vi "SMU Switch Handshaking - Advanced - DMM.vi"(4 "Source:Advanced:Source Delay":dbl=4e-05 format="%#_6p", 5 "Source:Transient Response":i32(ring)=1039 items=["Slow"=1041, "Normal"=1038, "Fast"=1039, "Custom"=1042], 7 "Measurement:Sense":i32(ring)=1008 items=["Local"=1008, "Remote"=1009], 8 "channels":string="0", 9 "Current":dbl=0.4 format="%#_6p", 10 "Voltage":dbl=0.6 format="%#_6p", 11 "resource name":refnum<k15>="SMU" caption="SMU resource name") -> ()   [LabVIEW 2019]
uses:
  <instrlib>/niSwitch/niSwitch.llb/niSwitch Topologies.ctl
  <instrlib>/niSwitch/niSwitch.llb/niSwitch Trigger Input.ctl
  <instrlib>/niSwitch/niSwitch.llb/niSwitch Scan Advanced Output.ctl
  <instrlib>/niDMM/nidmm.llb/niDMM Function.ctl
  <instrlib>/niDMM/nidmm.llb/niDMM Trigger.ctl
  <instrlib>/niDMM/nidmm.llb/niDMM Slope.ctl
  <instrlib>/niDCPower/nidcpower.llb/niDCPower Export Signal - Signal.ctl
  <instrlib>/niDMM/nidmm.llb/niDMM Sample Trigger.ctl
  <instrlib>/niDMM/nidmm.llb/niDMM Control Actions.ctl
  <instrlib>/niDCPower/nidcpower.llb/niDCPower Wait For Event - Event.ctl
  <instrlib>/niDCPower/nidcpower.llb/niDCPower Configure Digital Edge Start Trigger.vi
  <instrlib>/niDCPower/nidcpower.llb/niDCPower Configure Digital Edge Sequence Advance Trigger.vi
  <instrlib>/niDMM/nidmm.llb/niDMM Configure Measurement Absolute.vi
  <vilib>/ptbypt/NI_PtbyPt.lvlib
panel:
  out "R ch5":dbl=2.5910331699131763e-06 format="%#_8p"
  out "Waveform Chart ch5":dbl(graph)=2.5910331699131763e-06
  out "standard deviation ch5":dbl=1.2903874661428992e-07 format="%.6p"
  out "R ch2":dbl=7.972830555761924e-07 format="%#_8p"
  out "Waveform Chart ch2":dbl(graph)=7.972830555761924e-07
  out "standard deviation ch2":dbl=2.4873144111684715e-07 format="%.6p"
  out "R ch4":dbl=4.337850347432063e-06 format="%#_8p"
  out "Waveform Chart ch4":dbl(graph)=4.337850347432063e-06
  out "standard deviation ch4":dbl=1.3349477799504632e-07 format="%.6p"
  out "R ch1":dbl=1.766350792285936e-06 format="%#_8p"
  out "Waveform Chart ch1":dbl(graph)=1.766350792285936e-06
  out "standard deviation ch1":dbl=1.0073898391211356e-07 format="%.6p"
  out "R ch3":dbl=nan format="%#_8p"
  out "Waveform Chart ch3":dbl(graph)=nan
  out "standard deviation ch3":dbl=nan format="%.6p"
  out "standard deviation ch0":dbl=9.036112711225856e-08 format="%.6p"
  out "Waveform Chart ch0":dbl(graph)=2.086031872229756e-06
  out "R ch0":dbl=2.086031872229756e-06 format="%#_8p"
  out "voltage measurements":dbl[](array[numeric])=[1.0598444973016901e-05, 1.0214343256868734e-05, 1.0841159071034221e-05]
  in  "Configuration:Advanced:Number Of Averages":i32=1
  in  "Configuration:Advanced:Aperture Time":dbl=0.05
  in  "Configuration:Advanced:Aperture Time Units":i32(ring) items=["Seconds", "Power Line Cycles"]
  in  "Device Name":refnum<k15>="4082"
  in  "Slope":T1
  in  "DMM Trigger Source":T2=enum."TTL 2"
  in  "Range":dbl=0.1 format="%.2p"
  in  "Function":T3
  out "Elapsed Time (ms)":u32=9613
  in  "scan advanced output (External)":T4=enum."TTL1" caption="Scan Advanced Destination"
  in  "Trigger Source":T5=enum."TTL0"
  in  "topology name":T6="2530/1-Wire 4x32 Matrix" caption="Topology Name"
  in  "scan list":string="r0->c0&r1->c1&r2->c2&r3->c3;\nr0->c4&r1->c5&r2->c6&r3->c7;\nr0->c8&r1->c9&r2->c10&r3->c11;\nr0->c12&r1->c13&r2->c14&r3->c15;\nr0->c16&r1->c17&r2->c18&r3->c19;\nr0->c20&r1->c21&r2->c22&r3->c23;\n\n" caption="Scan List"
  in  "resource name 2":refnum<k15>="PXI1Slot5" caption="Switch Resource Name"
  in  "Measurement:Aperture Time":dbl=0.08333333 format="%#_6p"
  out "error out":errorcluster={"status"=FALSE, "code"=1073356801, "source"="niDMM Fetch Multi Point.vi<ERR>Over range.\n\n "}
  out "current measurements":dbl[](array[numeric])=[0.24066338808611681, -0.24109991223961136, -3.355526367182504e-08]
  in  "Measurement:Advanced:DC Noise Rejection":i32(ring)=1044 items=["Normal"=1044, "Second-Order"=1043]
  in  "Source:Advanced:Sequence Loop Count":i32=39
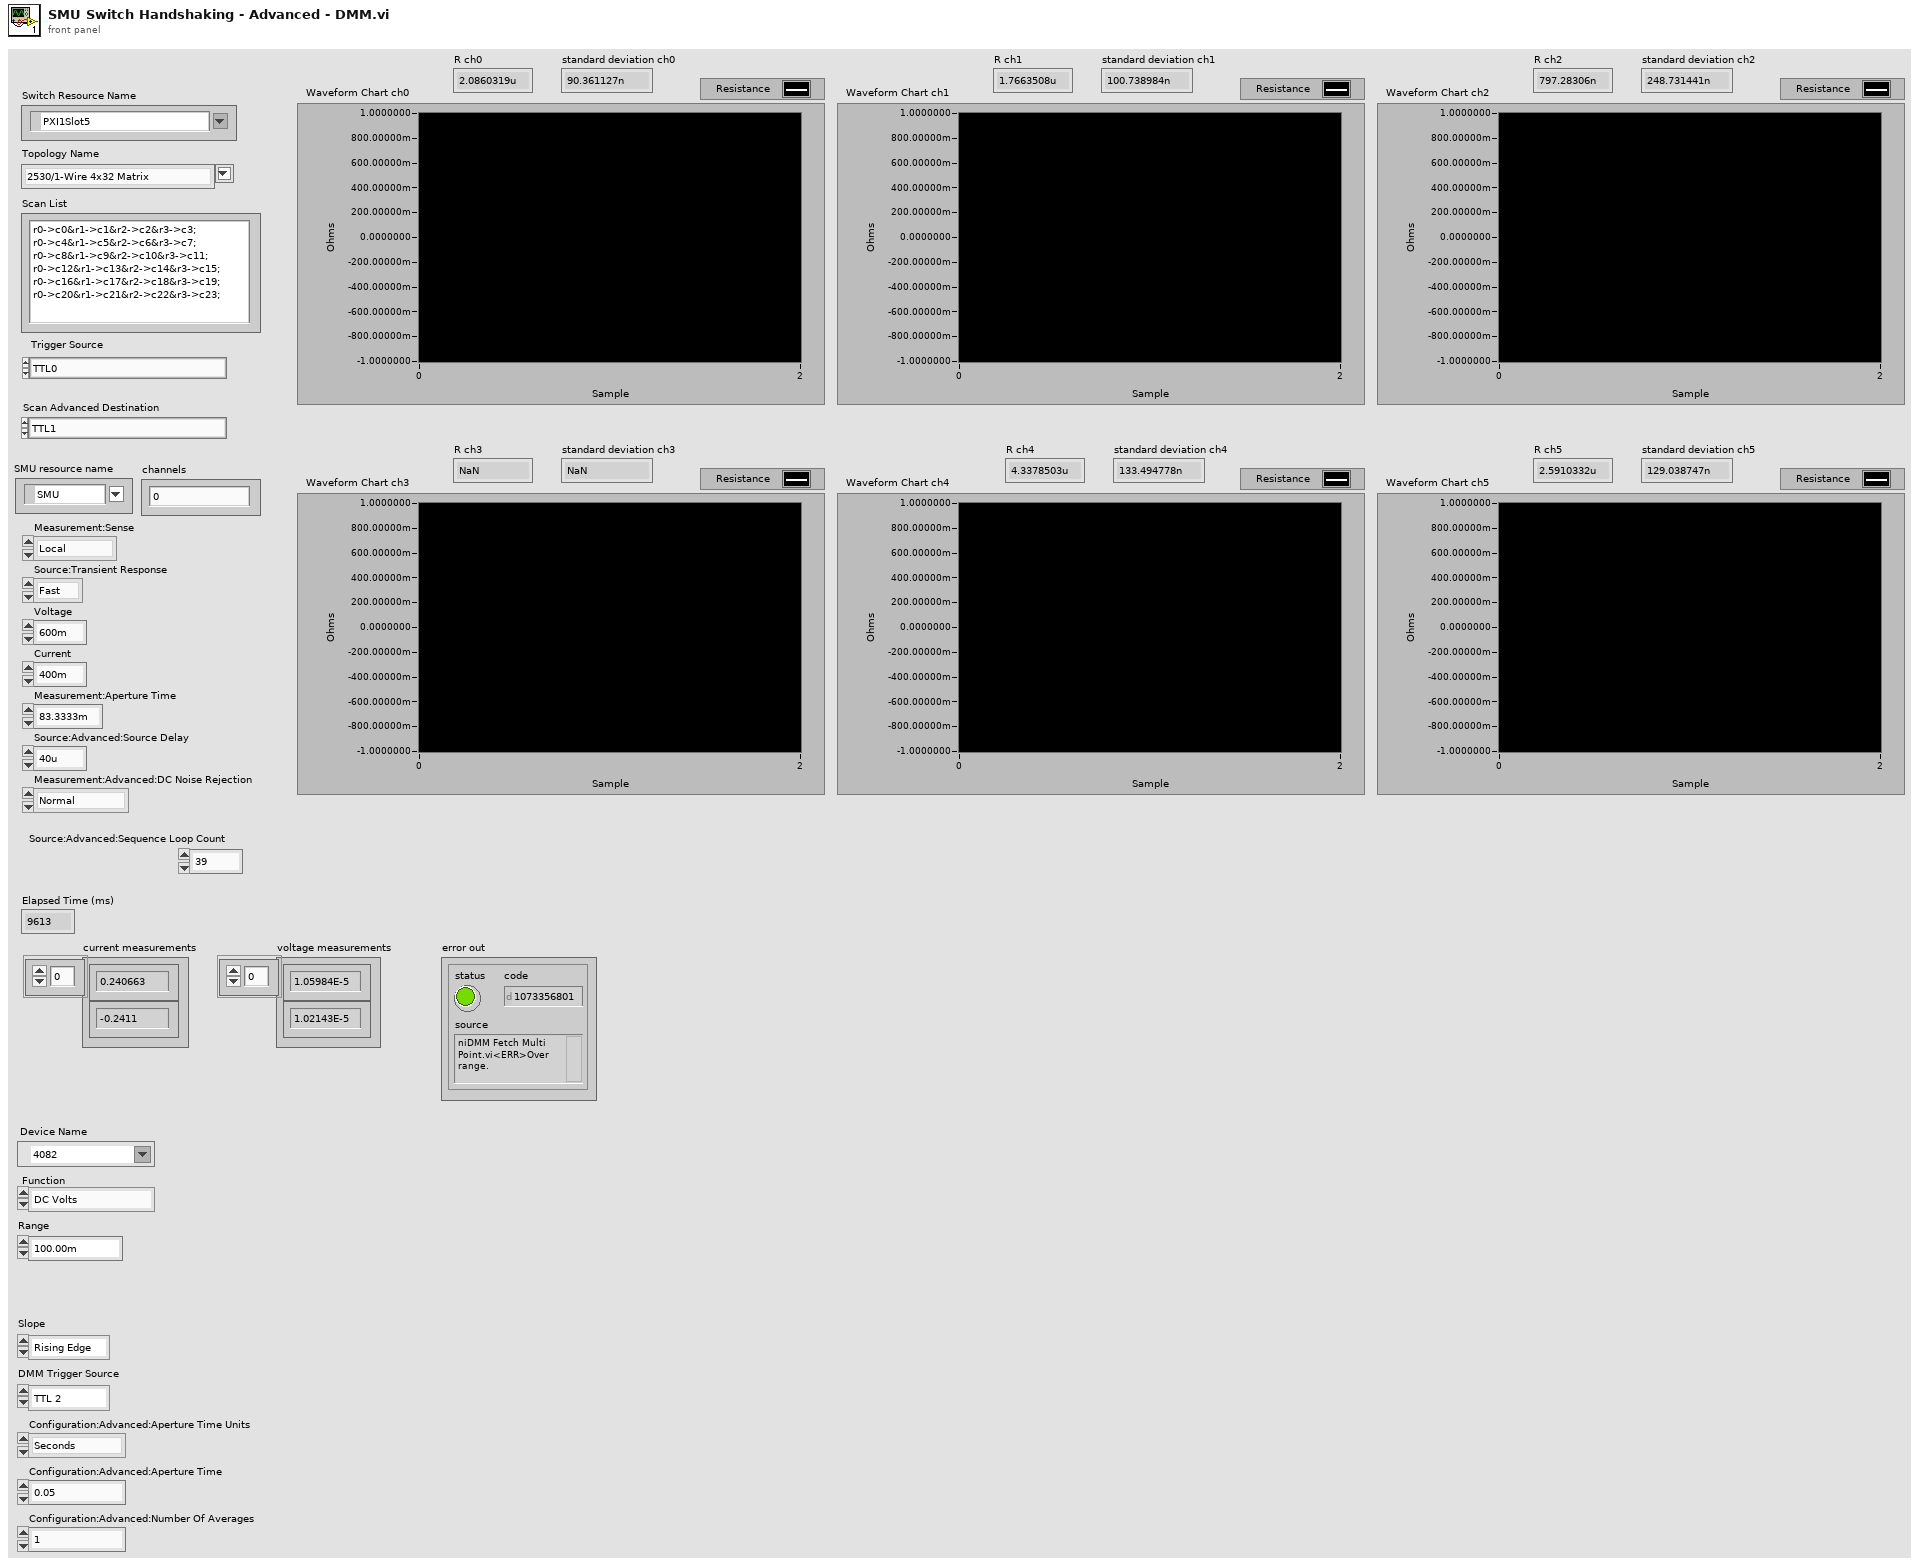
[diagram p1: front panel]
types:
  T1 = typedef "niDMM Slope.ctl" = enum16{"Rising Edge", "Falling Edge"}
  T2 = typedef "niDMM Trigger.ctl" = enum16{"Immediate", "External", "TTL 0", "TTL 1", "TTL 2", "TTL 3", "TTL 4", "TTL 5", "TTL 6", "Software", "TTL 7", "PXI Star", "LBR Trig 1", "Aux Trig 1"}
  T3 = typedef "niDMM Function.ctl" = enum16{"DC Volts", "AC Volts", "DC Current", "AC Current", "2-wire Resistance", "4-wire Resistance", "Diode", "Frequency", "Period", "AC Volts DC Coupled", "Capacitance", "Inductance", "Temperature"}
  T4 = typedef "niSwitch Scan Advanced Output.ctl" = enum16{"None", "External", "TTL0", "TTL1", "TTL2", "TTL3", "TTL4", "TTL5", "TTL6", "TTL7", "ECL0", "ECL1", "PXI Star", "Rear Connector", "Front Connector", "Rear Connector Module 1", "Rear Connector Module 2", "Rear Connector Module 3", "Rear Connector Module 4", "Rear Connector Module 5", "Rear Connector Module 6", "Rear Connector Module 7", "Rear Connector Module 8", "Rear Connector Module 9", "Rear Connector Module 10", "Rear Connector Module 11", "Rear Connector Module 12", "Front Connector Module 1", "Front Connector Module 2", "Front Connector Module 3", "Front Connector Module 4", "Front Connector Module 5", "Front Connector Module 6", "Front Connector Module 7", "Front Connector Module 8", "Front Connector Module 9", "Front Connector Module 10", "Front Connector Module 11", "Front Connector Module 12"}
  T5 = typedef "niSwitch Trigger Input.ctl" = enum16{"Immediate", "External", "TTL0", "TTL1", "TTL2", "TTL3", "TTL4", "TTL5", "TTL6", "TTL7", "ECL0", "ECL1", "PXI Star", "Software Trigger Function", "Rear Connector", "Front Connector", "Rear Connector of Module 1", "Rear Connector of Module 2", "Rear Connector of Module 3", "Rear Connector of Module 4", "Rear Connector of Module 5", "Rear Connector of Module 6", "Rear Connector of Module 7", "Rear Connector of Module 8", "Rear Connector of Module 9", "Rear Connector of Module 10", "Rear Connector of Module 11", "Rear Connector of Module 12", "Front Connector of Module 1", "Front Connector of Module 2", "Front Connector of Module 3", "Front Connector of Module 4", "Front Connector of Module 5", "Front Connector of Module 6", "Front Connector of Module 7", "Front Connector of Module 8", "Front Connector of Module 9", "Front Connector of Module 10", "Front Connector of Module 11", "Front Connector of Module 12"}
  T6 = typedef "niSwitch Topologies.ctl" = string
  T7 = typedef "niDCPower Export Signal - Signal.ctl" = i32
  T8 = typedef "niDMM Control Actions.ctl" = i32
  T9 = typedef "niDMM Sample Trigger.ctl" = enum16{"Immediate", "External", "TTL 0", "TTL 1", "TTL 2", "TTL 3", "TTL 4", "TTL 5", "TTL 6", "Interval", "Software", "TTL 7", "PXI Star", "LBR Trig 1", "Aux Trig 1"}
  T10 = typedef "niDCPower Wait For Event - Event.ctl" = i32
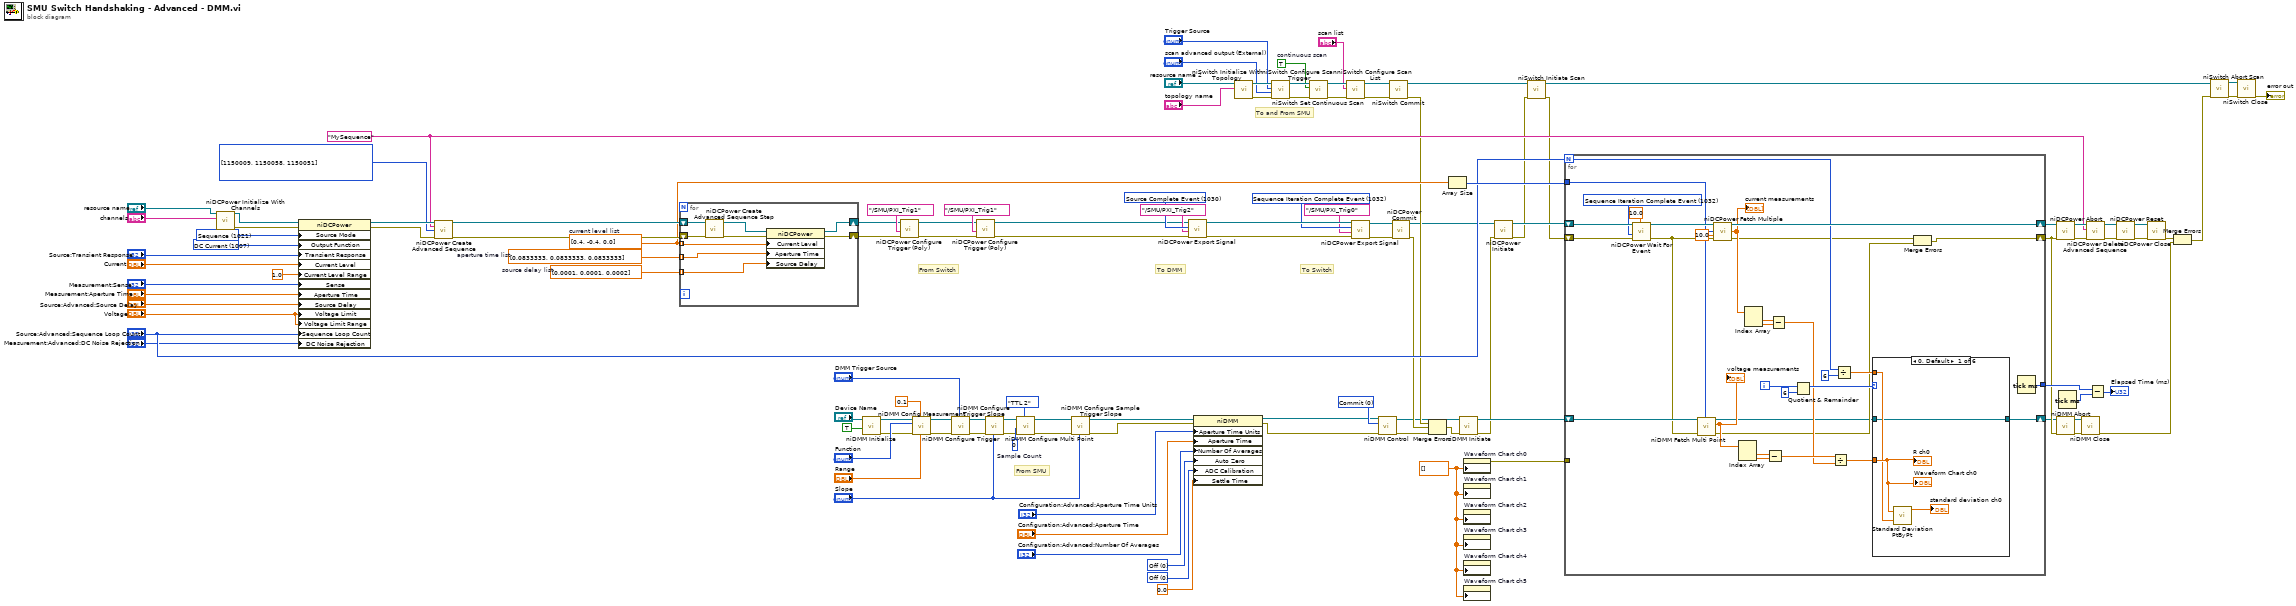
[diagram p0: block diagram]
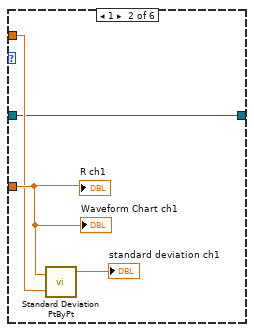
[diagram p2: hidden frame]
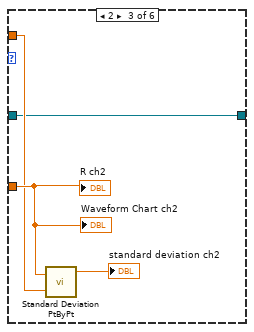
[diagram p3: hidden frame]
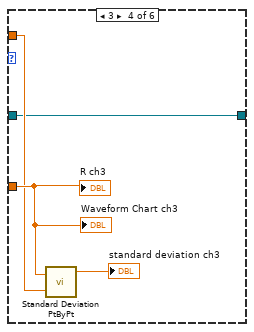
[diagram p4: hidden frame]
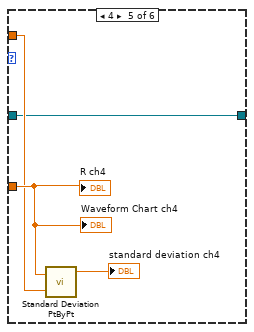
[diagram p5: hidden frame]
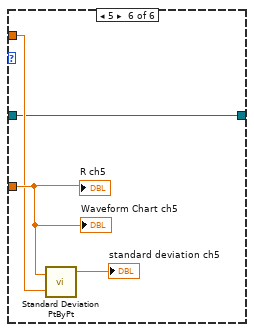
[diagram p6: hidden frame]
diagram:
  w2 = 0 items=["Auto"=-1, "Off"=0, "On"=1] ("Configuration:Measurement Options:ADC Calibration")
  w3 = 0 items=["Auto"=-1, "Off"=0, "On"=1, "Once"=2] ("Configuration:Measurement Options:Auto Zero")
  w7 = T7 1032 items=["Source Complete Event"=1030, "Measure Complete Event"=1031, "Sequence Iteration Complete Event"=1032, "Sequence Engine Done Event"=1033, "Pulse Complete Event"=1051, "Ready For Pulse Trigger Event"=1052, "Start Trigger"=1034, "Source Trigger"=1035, "Measure Trigger"=1036, "Sequence Advance Trigger"=1037, "Pulse Trigger"=1053] ("signal")
  w31 = T8 0 items=["Commit"] ("Control Action")
  w53 = 0  # Sample Count
  w58 = T7 1030 items=["Source Complete Event"=1030, "Measure Complete Event"=1031, "Sequence Iteration Complete Event"=1032, "Sequence Engine Done Event"=1033, "Pulse Complete Event"=1051, "Ready For Pulse Trigger Event"=1052, "Start Trigger"=1034, "Source Trigger"=1035, "Measure Trigger"=1036, "Sequence Advance Trigger"=1037, "Pulse Trigger"=1053] ("signal")
  w61 = dbl[] [0.4, -0.4, 0.0]  # current level list
  w8 = dbl[] [0.0833333, 0.0833333, 0.0833333]  # aperture time list
  w67 = i32[] [1150009, 1150058, 1150051] items=["Source -> Output Function"=1150008, "Source -> Output Enabled"=1250006, "Source -> Output Resistance"=1150061, "Source -> Transient Response"=1150062, "Source -> Custom Transient Response -> Voltage Gain Bandwidth"=1150067, "Source -> Custom Transient Response -> Voltage Compensation Frequency"=1150068, "Source -> Custom Transient Response -> Voltage Pole-Zero Ratio"=1150069, "Source -> Custom Transient Response -> Current Gain Bandwidth"=1150070, "Source -> Custom Transient Response -> Current Compensation Frequency"=1150071, "Source -> Custom Transient Response -> Current Pole-Zero Ratio"=1150072, "Source -> DC Voltage -> Voltage Level"=1250001, "Source -> DC Voltage -> Voltage Level Range"=1150005, "Source -> DC Voltage -> Current Limit"=1250005, "Source -> DC Voltage -> Current Limit High"=1150187, "Source -> DC Voltage -> Current Limit Low"=1150188, "Source -> DC Voltage -> Current Limit Range"=1150004, "Source -> DC Current -> Current Level"=1150009, "Source -> DC Current -> Current Level Range"=1150011, "Source -> DC Current -> Voltage Limit"=1150010, "Source -> DC Current -> Voltage Limit High"=1150185, "Source -> DC Current -> Voltage Limit Low"=1150186, "Source -> DC Current -> Voltage Limit Range"=1150012, "Source -> Pulse Voltage -> Pulse Voltage Level"=1150080, "Source -> Pulse Voltage -> Pulse Bias Voltage Level"=1150082, "Source -> Pulse Voltage -> Pulse Voltage Level Range"=1150084, "Source -> Pulse Voltage -> Pulse Current Limit"=1150081, "Source -> Pulse Voltage -> Pulse Current Limit High"=1150193, "Source -> Pulse Voltage -> Pulse Current Limit Low"=1150194, "Source -> Pulse Voltage -> Pulse Bias Current Limit"=1150083, "Source -> Pulse Voltage -> Pulse Bias Current Limit High"=1150195, "Source -> Pulse Voltage -> Pulse Bias Current Limit Low"=1150196, "Source -> Pulse Voltage -> Pulse Current Limit Range"=1150085, "Source -> Pulse Current -> Pulse Current Level"=1150086, "Source -> Pulse Current -> Pulse Bias Current Level"=1150088, "Source -> Pulse Current -> Pulse Current Level Range"=1150090, "Source -> Pulse Current -> Pulse Voltage Limit"=1150087, "Source -> Pulse Current -> Pulse Voltage Limit High"=1150189, "Source -> Pulse Current -> Pulse Voltage Limit Low"=1150190, "Source -> Pulse Current -> Pulse Bias Voltage Limit"=1150089, "Source -> Pulse Current -> Pulse Bias Voltage Limit High"=1150191, "Source -> Pulse Current -> Pulse Bias Voltage Limit Low"=1150192, "Source -> Pulse Current -> Pulse Voltage Limit Range"=1150091, "Source -> Advanced -> Source Delay"=1150051, "Source -> Advanced -> Pulse Bias Delay"=1150092, "Source -> Advanced -> Pulse On Time"=1150093, "Source -> Advanced -> Pulse Off Time"=1150094, "Source -> Advanced -> OVP Enabled"=1250002, "Source -> Advanced -> OVP Limit"=1250003, "Source -> Advanced -> Compliance Limit Symmetry"=1150184, "Source -> Advanced -> Sequence Step Delta Time"=1150198, "Measurement -> Sense"=1150013, "Measurement -> Aperture Time"=1150058, "Measurement -> Measure Record Length"=1150063, "Measurement -> Advanced -> DC Noise Rejection"=1150066] ("advanced sequence properties")
  w68 = "MySequence" ("sequence name")
  w100 = TRUE  # continuous scan
  w64 = dbl[] [0.0001, 0.0001, 0.0002]  # source delay list
  w11 = dbl[] [] ("History Data")
  w119 = 1007 items=["DC Voltage"=1006, "DC Current"=1007, "Pulse Voltage"=1049, "Pulse Current"=1050] ("Source:Output Function")
  w120 = 1021 items=["Single Point"=1020, "Sequence"=1021] ("Source:Source Mode")
  # "To and From SMU"
  # "From SMU"
  # "To Switch"
  # "To DMM"
  # "From Switch"
  n1 = call <instrlib>:"niDCPower Initialize With Channels.vi"("channels"="channels", "resource name"="resource name") -> ("error out"=w113:errorcluster, "instrument handle out"=w114:refnum<k15>)  [unwired: 8 in]
  n2 = property class="niDCPower"(reference=w114, error in=w113, "Source Mode"=w120, "Output Function"=w119, "Transient Response"="Source:Transient Response", "Current Level"="Current", "Current Level Range"=1.0 ("Source:DC Current:Current Level Range"), "Sense"="Measurement:Sense", "Aperture Time"="Measurement:Aperture Time", "Source Delay"="Source:Advanced:Source Delay", "Voltage Limit"="Voltage", "Voltage Limit Range"="Voltage", "Sequence Loop Count"="Source:Advanced:Sequence Loop Count", "DC Noise Rejection"="Measurement:Advanced:DC Noise Rejection") -> (reference out=w76:refnum<k15>, error out=w75:errorcluster)
  n3 = call <instrlib>:"niDCPower Create Advanced Sequence.vi"("instrument handle"=w76, "sequence name"=w68, "advanced sequence properties"=w67, "error in (no error)"=w75) -> ("instrument handle out"=w66:refnum<k15>, "error out"=w65:errorcluster)  [unwired: 10 in]
  n4 = for {
    shift-right: [w126] -> w62
    shift-left: w65 -> [w129]
    shift-right: [w125] -> w63
    shift-left: w66 -> [w124]
    tunnel: w64 -> [w123] mode=indexing
    tunnel: w61 -> [w121] mode=indexing
    tunnel: w8 -> [w122] mode=indexing
    n5 = call <instrlib>:"niDCPower Create Advanced Sequence Step.vi"("error in (no error)"=w129, "instrument handle"=w124) -> ("error out"=w127:errorcluster, "instrument handle out"=w128:refnum<k15>)  [unwired: 8 in]
    n6 = property class="niDCPower"(reference=w128, error in=w127, "Current Level"=w121, "Aperture Time"=w122, "Source Delay"=w123) -> (reference out=w125:refnum<k15>, error out=w126:errorcluster)
  }
  n7 = call <instrlib>:"niDMM Initialize.vi"("Reset"=TRUE, "Instrument Descriptor"="Device Name") -> ("error out"=w39:errorcluster, "instrument handle out"=w38:refnum<k15>)  [unwired: 8 in]
  n8 = call-poly <instrlib>:"niDCPower Configure Trigger (Poly).vi"("error in (no error)"=w62, "input terminal"=tag "/SMU/PXI_Trig1", "instrument handle"=w63) -> ("error out"=w81:errorcluster, "instrument handle out"=w82:refnum<k15>)  [unwired: 7 in]
  n9 = call-poly <instrlib>:"niDMM Config Measurement.vi"("Range"="Range", "Resolution"=0.1, "error in (no error)"=w39, "Function"="Function", "instrument handle"=w38) -> ("error out"=w45:errorcluster, "instrument handle out"=w44:refnum<k15>)  [unwired: 5 in]
  n10 = call <instrlib>:"niDMM Configure Trigger.vi"("Trigger Source"="DMM Trigger Source", "error in (no error)"=w45, "instrument handle"=w44) -> ("error out"=w47:errorcluster, "instrument handle out"=w46:refnum<k15>)  [unwired: 7 in]
  n11 = call-poly <instrlib>:"niDCPower Configure Trigger (Poly).vi"("error in (no error)"=w81, "input terminal"=tag "/SMU/PXI_Trig1", "instrument handle"=w82) -> ("error out"=w9:errorcluster, "instrument handle out"=w10:refnum<k15>)  [unwired: 7 in]
  n12 = call <instrlib>:"niDMM Configure Trigger Slope.vi"("Slope"="Slope", "error in (no error)"=w47, "instrument handle"=w46) -> ("error out"=w49:errorcluster, "instrument handle out"=w48:refnum<k15>)  [unwired: 7 in]
  n13 = call <instrlib>:"niDMM Configure Multi Point.vi"("Sample Trigger"=niDMM_Sample_Trigger."TTL 2", "error in (no error)"=w49, "Sample Count"=w53, "instrument handle"=w48) -> ("error out"=w51:errorcluster, "instrument handle out"=w50:refnum<k15>)  [unwired: 6 in]
  n14 = call <instrlib>:"niDMM Configure Sample Trigger Slope.vi"("Slope"="Slope", "error in (no error)"=w51, "instrument handle"=w50) -> ("error out"=w22:errorcluster, "instrument handle out"=w23:refnum<k15>)  [unwired: 7 in]
  n15 = call <instrlib>:"niDCPower Export Signal.vi"("error in (no error)"=w9, "output terminal"=tag "/SMU/PXI_Trig2", "signal"=w58, "instrument handle"=w10) -> ("error out"=w59:errorcluster, "instrument handle out"=w60:refnum<k15>)  [unwired: 6 in]
  n16 = property class="niDMM"(reference=w23, error in=w22, "Aperture Time Units"="Configuration:Advanced:Aperture Time Units", "Aperture Time"="Configuration:Advanced:Aperture Time", "Number Of Averages"="Configuration:Advanced:Number Of Averages", "Auto Zero"=w3, "ADC Calibration"=w2, "Settle Time"=0.0 ("Configuration:Advanced:Settle Time")) -> (reference out=w13:refnum<k15>, error out=w12:errorcluster)
  n17 = call <instrlib>:"niSwitch Initialize With Topology.vi"("topology name"="topology name", "resource name"="resource name 2") -> ("error out"=w97:errorcluster, "instrument handle out"=w98:refnum<k15>)  [unwired: 3 in, 5 out]
  n18 = call <instrlib>:"niSwitch Configure Scan Trigger.vi"("error in (no error)"=w97, "scan advanced output (External)"="scan advanced output (External)", "trigger input (External)"="Trigger Source", "instrument handle"=w98) -> ("error out"=w101:errorcluster, "instrument handle out"=w103:refnum<k15>)  [unwired: 1 in, 5 out]
  n19 = call <instrlib>:"niSwitch Set Continuous Scan.vi"("error in (no error)"=w101, "continuous scan (False)"=w100, "instrument handle"=w103) -> ("error out"=w95:errorcluster, "instrument handle out"=w96:refnum<k15>)  [unwired: 7 out]
  n20 = call <instrlib>:"niSwitch Configure Scan List.vi"("error in (no error)"=w95, "scan list"="scan list", "instrument handle"=w96) -> ("error out"=w92:errorcluster, "instrument handle out"=w91:refnum<k15>)  [unwired: 1 in, 6 out]
  n21 = call <instrlib>:"niDCPower Export Signal.vi"("error in (no error)"=w59, "output terminal"=tag "/SMU/PXI_Trig0", "signal"=w7, "instrument handle"=w60) -> ("error out"=w34:errorcluster, "instrument handle out"=w35:refnum<k15>)  [unwired: 6 in]
  n22 = call <instrlib>:"niDMM Control.vi"("error in (no error)"=w12, "Control Action"=w31, "instrument handle"=w13) -> ("error out"=w30:errorcluster, "instrument handle out"=w24:refnum<k15>)  [unwired: 7 in]
  n23 = call <instrlib>:"niSwitch Commit.vi"("error in (no error)"=w92, "instrument handle"=w91) -> ("error out"=w33:errorcluster, "instrument handle out"=w90:refnum<k15>)  [unwired: 8 out]
  n24 = call <instrlib>:"niDCPower Commit.vi"("error in (no error)"=w34, "instrument handle"=w35) -> ("error out"=w32:errorcluster, "instrument handle out"=w27:refnum<k15>)  [unwired: 8 in]
  n25 = Merge Errors(w33, w32, w30) -> (w29:errorcluster)
  n26 = Array Size(array=w61) -> (size(s)=w115:i32)
  n27 = call <instrlib>:"niDMM Initiate.vi"("error in (no error)"=w29, "instrument handle"=w24) -> ("error out"=w28:errorcluster, "instrument handle out"=w36:refnum<k15>)  [unwired: 8 in]
  n28 = property on="Waveform Chart ch0" class="WFChart (strict)"("History Data"=w11) -> (error out=w5:errorcluster)  [unwired: 2 in, 1 out]
  n29 = property on="Waveform Chart ch1" class="WFChart (strict)"("History Data"=w11) -> ()  [unwired: 2 in, 2 out]
  n30 = property on="Waveform Chart ch2" class="WFChart (strict)"("History Data"=w11) -> ()  [unwired: 2 in, 2 out]
  n31 = property on="Waveform Chart ch3" class="WFChart (strict)"("History Data"=w11) -> ()  [unwired: 2 in, 2 out]
  n32 = property on="Waveform Chart ch4" class="WFChart (strict)"("History Data"=w11) -> ()  [unwired: 2 in, 2 out]
  n33 = property on="Waveform Chart ch5" class="WFChart (strict)"("History Data"=w11) -> ()  [unwired: 2 in, 2 out]
  n34 = call <instrlib>:"niDCPower Initiate.vi"("error in (no error)"=w28, "instrument handle"=w27) -> ("error out"=w26:errorcluster, "instrument handle out"=w104:refnum<k15>)  [unwired: 8 in]
  n35 = call <instrlib>:"niSwitch Initiate Scan.vi"("error in (no error)"=w26, "instrument handle"=w90) -> ("error out"=w25:errorcluster, "instrument handle out"=w93:refnum<k15>)  [unwired: 8 out]
  n36 = for {
    N: "Source:Advanced:Sequence Loop Count" -> [w149]
    tunnel: w115 -> [w143]
    shift-right: [w134] -> w18
    shift-left: w25 -> [w145]
    shift-right: [w156] -> w108
    shift-left: w104 -> [w160]
    tunnel: w5 -> [_]
    tunnel: [w153] -> w80
    shift-right: [w132] -> w14
    shift-left: w36 -> [w144]
    i -> [w152]
    w159 = T10 1032 items=["Source Complete Event"=1030, "Measure Complete Event"=1031, "Sequence Iteration Complete Event"=1032, "Sequence Engine Done Event"=1033, "Pulse Complete Event"=1051, "Ready For Pulse Trigger Event"=1052] ("event")
    n37 = call <instrlib>:"niDCPower Wait For Event.vi"("timeout (sec)"=10.0, "error in (no error)"=w145, "event"=w159, "instrument handle"=w160) -> ("error out"=w131:errorcluster, "instrument handle out"=w157:refnum<k15>)  [unwired: 6 in]
    n38 = call <instrlib>:"niDMM Fetch Multi Point.vi"("Number to Fetch"=w143, "error in (no error)"=w131, "instrument handle"=w144) -> ("error out"=w135:errorcluster, "Measurements"=w137:dbl[], "instrument handle out"=w133:refnum<k15>)  [unwired: 5 in, 1 out]
    "voltage measurements" <- w137
    n39 = call <instrlib>:"niDCPower Fetch Multiple.vi"("instrument handle"=w157, "count (1)"=w143, "timeout (sec)"=10.0, "error in (no error)"=w131) -> ("instrument handle out"=w156:refnum<k15>, "current measurements"=w155:dbl[], "error out"=w136:errorcluster)  [unwired: 6 in, 3 out]
    "current measurements" <- w155
    n40 = Index Array(array=w137) -> (element #1=w142:dbl, element #2=w141:dbl)  [unwired: 2 in]
    n41 = Index Array(array=w155) -> (element #1=w154:dbl, element #2=w146:dbl)  [unwired: 2 in]
    n42 = Subtract(x=w142, y=w141) -> (x-y=w140:dbl)
    n43 = Subtract(x=w154, y=w146) -> (x-y=w139:dbl)
    n44 = Quotient & Remainder(x=w152, y=6) -> (x-y*floor(x/y)=w150:i32)  [unwired: 1 out]
    n45 = Divide(x=w140, y=w139) -> (x/y=w138:dbl)
    n46 = Divide(x=w149, y=6) -> (x/y=w147:dbl)
    n47 = case shown="0, Default" w150 {
      tunnel: w147 -> [w162 w166 w170 w174 w178 w182]
      tunnel: w138 -> [w163 w167 w171 w175 w179 w183]
      tunnel: w133 -> [w161 w165 w169 w173 w177 w181]
      tunnel: [w161 w165 w169 w173 w177 w181] -> w132
      frame 0, Default {
        n48 = call <vilib>:"Standard Deviation PtByPt.vi"("x"=w163, "sample length"=w162) -> ("standard deviation"=→"standard deviation ch0":dbl)  [unwired: 1 in, 2 out]
        "R ch0" <- w163
        "Waveform Chart ch0" <- w163
      }
      frame 1 {
        n49 = call <vilib>:"Standard Deviation PtByPt.vi"("x"=w167, "sample length"=w166) -> ("standard deviation"=→"standard deviation ch1":dbl)  [unwired: 1 in, 2 out]
        "R ch1" <- w167
        "Waveform Chart ch1" <- w167
      }
      frame 2 {
        n50 = call <vilib>:"Standard Deviation PtByPt.vi"("x"=w171, "sample length"=w170) -> ("standard deviation"=→"standard deviation ch2":dbl)  [unwired: 1 in, 2 out]
        "R ch2" <- w171
        "Waveform Chart ch2" <- w171
      }
      frame 3 {
        n51 = call <vilib>:"Standard Deviation PtByPt.vi"("x"=w175, "sample length"=w174) -> ("standard deviation"=→"standard deviation ch3":dbl)  [unwired: 1 in, 2 out]
        "R ch3" <- w175
        "Waveform Chart ch3" <- w175
      }
      frame 4 {
        n52 = call <vilib>:"Standard Deviation PtByPt.vi"("x"=w179, "sample length"=w178) -> ("standard deviation"=→"standard deviation ch4":dbl)  [unwired: 1 in, 2 out]
        "R ch4" <- w179
        "Waveform Chart ch4" <- w179
      }
      frame 5 {
        n53 = call <vilib>:"Standard Deviation PtByPt.vi"("x"=w183, "sample length"=w182) -> ("standard deviation"=→"standard deviation ch5":dbl)  [unwired: 1 in, 2 out]
        "R ch5" <- w183
        "Waveform Chart ch5" <- w183
      }
    }
    n54 = Merge Errors(w136, w135) -> (w134:errorcluster)
    n55 = Tick Count (ms)() -> (millisecond timer value=w153:u32)
  }
  n56 = call <instrlib>:"niDCPower Abort.vi"("error in (no error)"=w18, "instrument handle"=w108) -> ("error out"=w73:errorcluster, "instrument handle out"=w74:refnum<k15>)  [unwired: 8 in]
  n57 = call <instrlib>:"niDMM Abort.vi"("error in (no error)"=w18, "instrument handle"=w14) -> ("error out"=w41:errorcluster, "instrument handle out"=w40:refnum<k15>)  [unwired: 8 in]
  n58 = Tick Count (ms)() -> (millisecond timer value=w79:u32)
  n59 = call <instrlib>:"niDMM Close.vi"("error in (no error)"=w41, "instrument handle"=w40) -> ("error out"=w17:errorcluster)  [unwired: 9 in]
  n60 = call <instrlib>:"niDCPower Delete Advanced Sequence.vi"("error in (no error)"=w73, "sequence name"=w68, "instrument handle"=w74) -> ("error out"=w72:errorcluster, "instrument handle out"=w71:refnum<k15>)  [unwired: 7 in]
  n61 = Subtract(x=w80, y=w79) -> (x-y=→"Elapsed Time (ms)":u32)
  n62 = call <instrlib>:"niDCPower Reset.vi"("error in (no error)"=w72, "instrument handle"=w71) -> ("error out"=w69:errorcluster, "instrument handle out"=w70:refnum<k15>)  [unwired: 2 in, 6 out]
  n63 = call <instrlib>:"niDCPower Close.vi"("error in (no error)"=w69, "instrument handle"=w70) -> ("error out"=w16:errorcluster)  [unwired: 9 in]
  n64 = Merge Errors(w16, w17) -> (w15:errorcluster)
  n65 = call <instrlib>:"niSwitch Abort Scan.vi"("error in (no error)"=w15, "instrument handle"=w93) -> ("error out"=w99:errorcluster, "instrument handle out"=w102:refnum<k15>)  [unwired: 8 out]
  n66 = call <instrlib>:"niSwitch Close.vi"("error in (no error)"=w99, "instrument handle"=w102) -> ("error out"=→"error out":errorcluster)  [unwired: 9 out]
